vi "test.vi"() -> ()   [LabVIEW 2010]
uses:
  <vilib>/Utility/miscctls.llb/LVRectTypeDef.ctl
panel:
  out "output cluster":T1
  out "Front Panel Window:Panel Bounds":T1
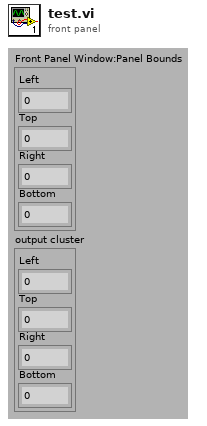
[diagram p1: front panel]
types:
  T1 = typedef "LVRectTypeDef.ctl" = cluster{"Left":i16, "Top":i16, "Right":i16, "Bottom":i16}
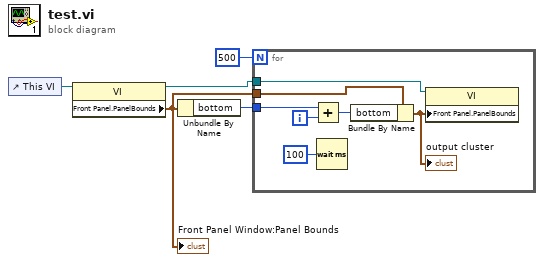
[diagram p0: block diagram]
diagram:
  n1 = control-ref of="This VI"() -> (w5:refnum<vi>)
  n2 = property class="VI"(reference=w5) -> (reference out=w4:refnum<vi>, "Front Panel.PanelBounds"=w3:T1)  [unwired: 1 in, 1 out]
  "Front Panel Window:Panel Bounds" <- w3
  n3 = Unbundle By Name(w3) -> ("bottom"=w2:i16)
  n4 = for {
    N: 500 -> [_]
    tunnel: w4 -> [w11]
    tunnel: w3 -> [w10]
    tunnel: w2 -> [w8]
    i -> [w7]
    n5 = Add(x=w8, y=w7) -> (x+y=w9:i32)
    n6 = Wait (ms)(milliseconds to wait=u32 100) -> ()  [unwired: 1 out]
    n7 = Bundle By Name(cluster=w10, "bottom"=w9) -> (w12:T1)
    "output cluster" <- w12
    n8 = property class="VI"(reference=w11, "Front Panel.PanelBounds"=w12) -> ()  [unwired: 1 in, 2 out]
  }
